vi "2D_Jacobi_eigenvalue_algorithm_v2.vi"() -> (3 "Jacobi Eigvals":dbl[](array[numeric]))   [LabVIEW 2020]
uses:
  <vilib>/Analysis/baseanly.llb/Real A x B.vi
  <vilib>/Analysis/Matrix/Numeric/Conversions/Array To Matrix - RA2.vi
  <vilib>/Analysis/Matrix/Numeric/Conversions/Matrix To Array - RM.vi
  <vilib>/Analysis/7linalg.llb/Real Eigenvalues and Vectors.vi
  <vilib>/Analysis/Matrix/NI_Matrix.lvlib
  <vilib>/Analysis/NI_AALBase.lvlib
  <vilib>/Analysis/NI_AALPro.lvlib
panel:
  out "A":dbl[][](array[numeric])
  out "summ of error":dbl
  out "LabVIEW eigvals":dbl[](array[numeric])
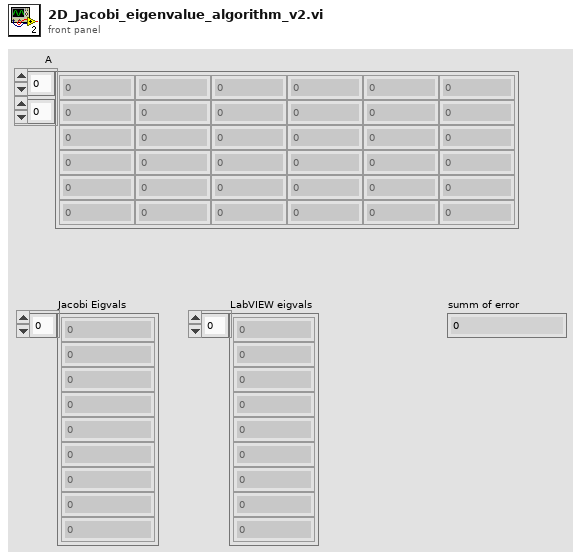
[diagram p1: front panel]
types:
  T1 = typedef "NI_Matrix.lvlib/RealMatrix.ctl" = dbl[][]
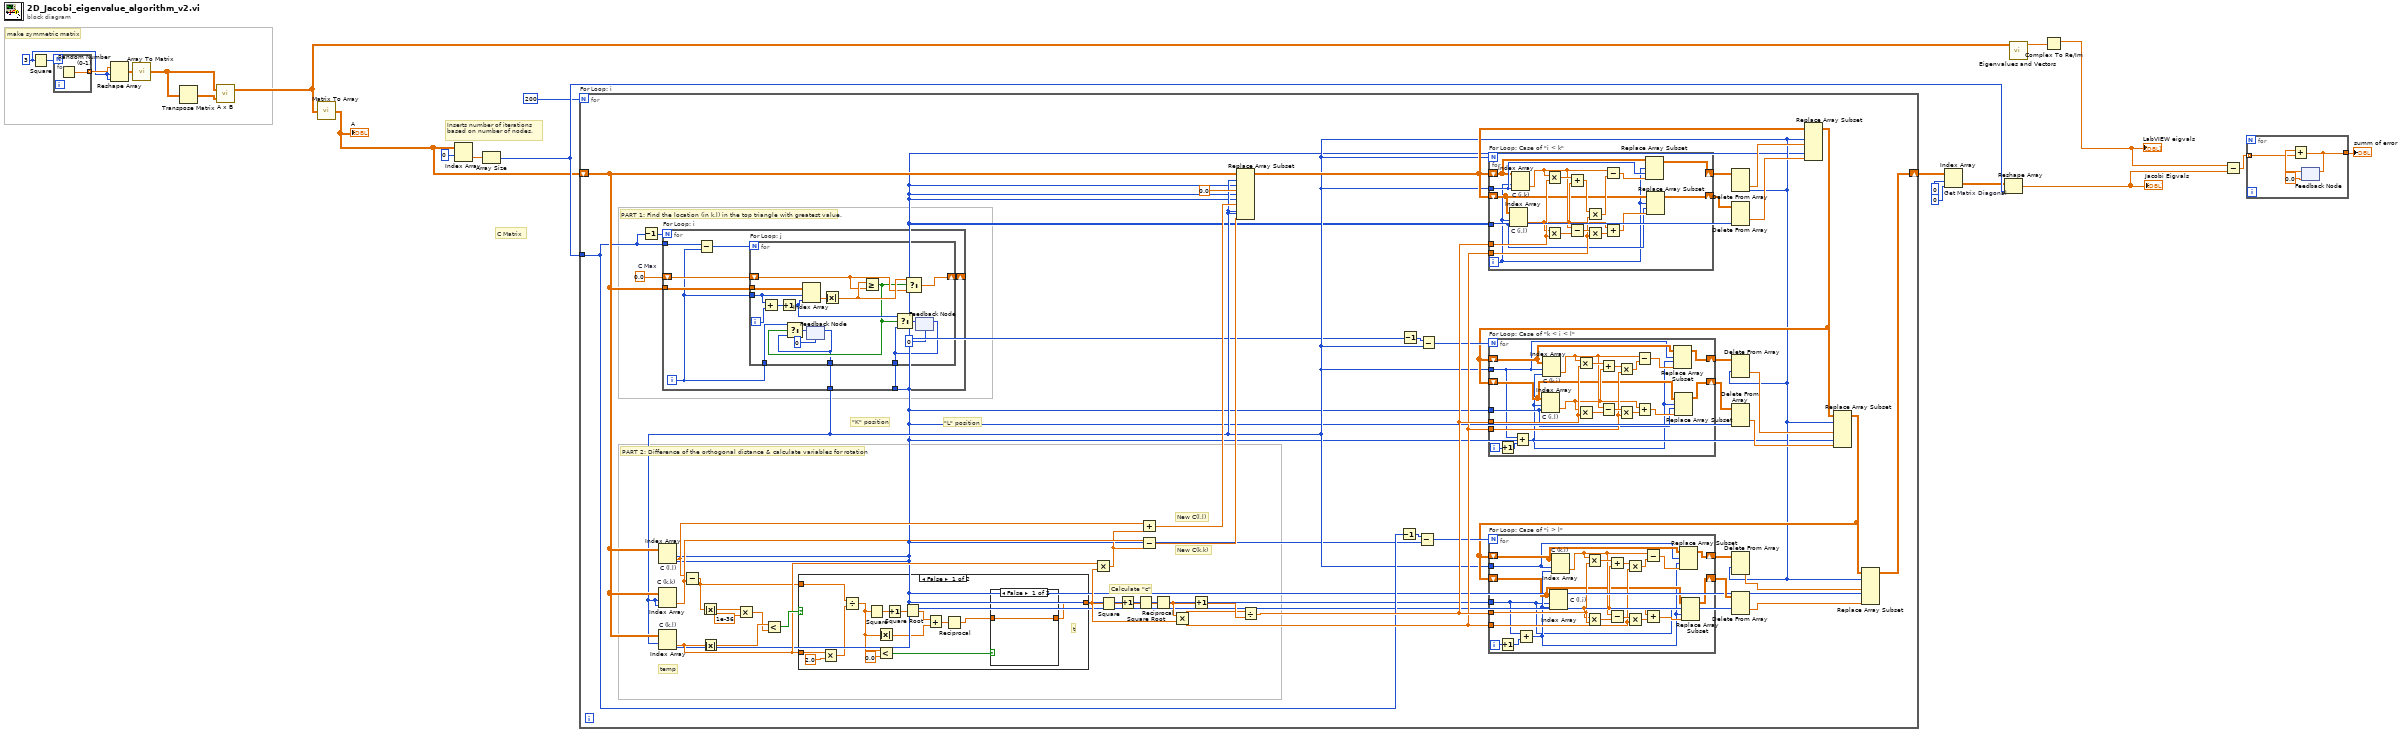
[diagram p0: block diagram]
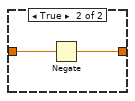
[diagram p2: hidden frame]
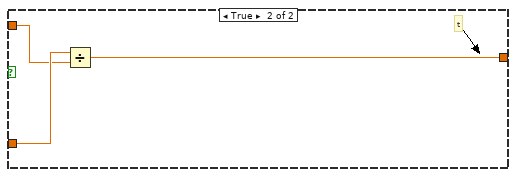
[diagram p3: hidden frame]
diagram:
  w11 = 3 ("x")
  # "make symmetric matrix"
  # "C Matrix"
  # "Inserts number of iterations\nbased on number of nodes."
  n1 = Square(x=w11) -> (x^2=w13:i32)
  n2 = for {
    N: w13 -> [_]
    tunnel: [w22] -> w12 mode=indexing
    n3 = Random Number (0-1)() -> (number: 0 to 1=w22:dbl)
  }
  n4 = Reshape Array(w12, w11, w11) -> (w10:dbl[][])
  n5 = call-poly <vilib>:"Array To Matrix.vi"("Real 2D Array"=w10) -> ("Real Matrix"=w9:T1)
  n6 = Transpose Matrix(1:w9) -> (0:w8:T1)
  n7 = call-poly <vilib>:"A x B.vi"("B"=w8, "A"=w9) -> ("A x B"=w2:T1)  [unwired: 1 out]
  n8 = call-poly <vilib>:"Matrix To Array.vi"("Real Matrix"=w2) -> ("Real 2D Array"=w1:dbl[][])
  "A" <- w1
  n9 = Index Array(array=w1, index (row)=0) -> (element=w14:dbl[])  [unwired: 1 in]
  n10 = Array Size(array=w14) -> (size(s)=w20:i32)
  n11 = for "For Loop: i" {
    N: 200 ("Max Rotation") -> [_]
    tunnel: w20 -> [w25]
    shift-right: [w29] -> w21
    shift-left: w1 -> [w47]
    w68 = 0.0  # C Max
    # "\"L\" position"
    # "\"K\" position"
    # "PART 2: Difference of the orthogonal distance & calculate variables for rotation"
    # "PART 1: Find the location (in k,l) in the top triangle with greatest value."
    # "New C(l,l)"
    # "New C(k,k)"
    # "temp"
    # "Calculate \"c\""
    n12 = Decrement(x=w25) -> (x-1=w69:i32)
    n13 = for "For Loop: i" {
      N: w69 -> [_]
      tunnel: w47 -> [w158]
      tunnel: w25 -> [w151]
      shift-right: [w156] -> _
      shift-left: w68 -> [w154]
      tunnel: [w155] -> w23
      tunnel: [w153] -> w24
      i -> [w152]
      n14 = Subtract(x=w151, y=w152) -> (x-y=w157:i32)
      n15 = for "For Loop: j" {
        N: w157 -> [_]
        tunnel: w158 -> [w174]
        tunnel: w152 -> [w171]
        shift-right: [w168] -> w156
        shift-left: w154 -> [w169]
        tunnel: [w165] -> w155
        tunnel: [w162] -> w153
        tunnel: w152 -> [w161]
        i -> [w173]
        n16 = Add(x=w171, y=w173) -> (x+y=w172:i32)
        n17 = Increment(x=w172) -> (x+1=w167:i32)
        n18 = Index Array(array=w174, index (row)=w171, index (col)=w167) -> (element=w175:dbl)
        n19 = feedback #1(0) -> (w162:i32)
        n20 = Absolute Value(x=w175) -> (abs(x)=w170:dbl)
        n21 = Greater Or Equal?(x=w170, y=w169) -> (x >= y?=w163:bool)
        n22 = Select(t=w161, s=w163, f=w162) -> (s? t:f=w164:i32)
        n23 = feedback-in #1(w164) -> ()
        n24 = Select(t=w170, s=w163, f=w169) -> (s? t:f=w168:dbl)
        n25 = feedback #2(0) -> (w165:i32)
        n26 = Select(t=w167, s=w163, f=w165) -> (s? t:f=w166:i32)
        n27 = feedback-in #2(w166) -> ()
      }
    }
    n28 = Index Array "C (l,l)"(array=w47, index (row)=w23, index (col)=w23) -> (element=w53:dbl)
    n29 = Index Array "C (k,k)"(array=w47, index (row)=w24, index (col)=w24) -> (element=w57:dbl)
    n30 = Index Array "C (k,l)"(array=w47, index (row)=w24, index (col)=w23) -> (element=w56:dbl)
    n31 = Subtract(x=w53, y=w57) -> (x-y=w48:dbl)
    n32 = Absolute Value(x=w48) -> (abs(x)=w65:dbl)
    n33 = Absolute Value(x=w56) -> (abs(x)=w67:dbl)
    n34 = Multiply(x=w65, y=1e-36 ("x")) -> (x*y=w66:dbl)
    n35 = Less?(x=w67, y=w66) -> (x < y?=w63:bool)
    n36 = case shown="False" w63 {
      tunnel: w56 -> [w144 w150]
      tunnel: w48 -> [w141 w149]
      tunnel: [w131 w148] -> w55
      frame False {
        # "t"
        n37 = Multiply(x=w144, y=2.0) -> (x*y=w142:dbl)
        n38 = Divide(x=w141, y=w142) -> (x/y=w135:dbl)
        n39 = Square(x=w135) -> (x^2=w139:dbl)
        n40 = Absolute Value(x=w135) -> (abs(x)=w140:dbl)
        n41 = Less?(x=w135, y=0.0) -> (x < y?=w133:bool)
        n42 = Increment(x=w139) -> (x+1=w138:dbl)
        n43 = Square Root(x=w138) -> (sqrt(x)=w137:dbl)
        n44 = Add(x=w137, y=w140) -> (x+y=w136:dbl)
        n45 = Reciprocal(x=w136) -> (1/x=w132:dbl)
        n46 = case shown="False" w133 {
          tunnel: w132 -> [w145 w147]
          tunnel: [w145 w146] -> w131
          frame False {
          }
          frame True {
            n47 = Negate(x=w147) -> (-x=w146:dbl)
          }
        }
      }
      frame True {
        # "t"
        n48 = Divide(x=w150, y=w149) -> (x/y=w148:dbl)
      }
    }
    n49 = Multiply(x=w56, y=w55) -> (x*y=w54:dbl)
    n50 = Square(x=w55) -> (x^2=w62:dbl)
    n51 = Increment(x=w62) -> (x+1=w61:dbl)
    n52 = Square Root(x=w61) -> (sqrt(x)=w60:dbl)
    n53 = Add(x=w53, y=w54) -> (x+y=w45:dbl)
    n54 = Subtract(x=w57, y=w54) -> (x-y=w46:dbl)
    n55 = Reciprocal(x=w60) -> (1/x=w59:dbl)
    n56 = Multiply(x=w59, y=w55) -> (x*y=w51:dbl)
    n57 = Increment(x=w59) -> (x+1=w58:dbl)
    n58 = Replace Array Subset(array=w47, new element #1=0.0 ("new element/subarray"), index (row) #1=w24, index (col) #1=w23, new element #2=w45, index (row) #2=w23, index (col) #2=w23, new element #3=w46, index (row) #3=w24, index (col) #3=w24) -> (w40:dbl[][])
    n59 = Divide(x=w51, y=w58) -> (x/y=w52:dbl)
    n60 = Decrement(x=w25) -> (x-1=w26:i32)
    n61 = Decrement(x=w23) -> (x-1=w27:i32)
    n62 = Subtract(x=w26, y=w23) -> (x-y=w50:i32)
    n63 = Subtract(x=w27, y=w24) -> (x-y=w49:i32)
    n64 = for "For Loop: Case of \"i < k\"" {
      N: w24 -> [_]
      tunnel: w52 -> [w127]
      tunnel: w51 -> [w124]
      tunnel: w24 -> [w119]
      tunnel: w23 -> [w114]
      shift-right: [w117] -> w44
      shift-left: w40 -> [w118]
      shift-right: [w113] -> w43
      shift-left: w40 -> [w116]
      i -> [w112]
      n65 = Index Array "C (i,l)"(array=w116, index (row)=w112, index (col)=w114) -> (element=w121:dbl)
      n66 = Index Array "C (i,k)"(array=w118, index (row)=w112, index (col)=w119) -> (element=w122:dbl)
      n67 = Multiply(x=w122, y=w127) -> (x*y=w130:dbl)
      n68 = Multiply(x=w121, y=w127) -> (x*y=w126:dbl)
      n69 = Add(x=w130, y=w121) -> (x+y=w129:dbl)
      n70 = Subtract(x=w122, y=w126) -> (x-y=w125:dbl)
      n71 = Multiply(x=w129, y=w124) -> (x*y=w128:dbl)
      n72 = Multiply(x=w125, y=w124) -> (x*y=w123:dbl)
      n73 = Subtract(x=w122, y=w128) -> (x-y=w120:dbl)
      n74 = Add(x=w121, y=w123) -> (x+y=w115:dbl)
      n75 = Replace Array Subset(array=w118, new element=w120, index (row)=w112, index (col)=w119) -> (w117:dbl[][])
      n76 = Replace Array Subset(array=w116, new element=w115, index (row)=w112, index (col)=w114) -> (w113:dbl[][])
    }
    n77 = Delete From Array(array=w44, index (col)=w24) -> (deleted portion=w41:dbl[])  [unwired: 2 in, 1 out]
    n78 = Delete From Array(array=w43, index (col)=w23) -> (deleted portion=w42:dbl[])  [unwired: 2 in, 1 out]
    n79 = Replace Array Subset(array=w40, new element #1=w41, index (col) #1=w24, new element #2=w42, index (col) #2=w23) -> (w37:dbl[][])  [unwired: 2 in]
    n80 = for "For Loop: Case of \"k < i < l\"" {
      N: w49 -> [_]
      tunnel: w52 -> [w108]
      tunnel: w51 -> [w105]
      tunnel: w23 -> [w95]
      tunnel: w24 -> [w93]
      shift-right: [w99] -> w36
      shift-left: w37 -> [w101]
      shift-right: [w98] -> w35
      shift-left: w37 -> [w97]
      i -> [w92]
      n81 = Increment(x=w92) -> (x+1=w91:i32)
      n82 = Add(x=w93, y=w91) -> (x+y=w94:i32)
      n83 = Index Array "C (i,l)"(array=w97, index (row)=w94, index (col)=w95) -> (element=w102:dbl)
      n84 = Index Array "C (k,i)"(array=w101, index (row)=w93, index (col)=w94) -> (element=w103:dbl)
      n85 = Multiply(x=w103, y=w108) -> (x*y=w111:dbl)
      n86 = Multiply(x=w102, y=w108) -> (x*y=w107:dbl)
      n87 = Add(x=w111, y=w102) -> (x+y=w110:dbl)
      n88 = Subtract(x=w103, y=w107) -> (x-y=w106:dbl)
      n89 = Multiply(x=w110, y=w105) -> (x*y=w109:dbl)
      n90 = Multiply(x=w106, y=w105) -> (x*y=w104:dbl)
      n91 = Subtract(x=w103, y=w109) -> (x-y=w100:dbl)
      n92 = Add(x=w102, y=w104) -> (x+y=w96:dbl)
      n93 = Replace Array Subset(array=w101, new element=w100, index (row)=w93, index (col)=w94) -> (w99:dbl[][])
      n94 = Replace Array Subset(array=w97, new element=w96, index (row)=w94, index (col)=w95) -> (w98:dbl[][])
    }
    n95 = Delete From Array(array=w36, index (row)=w24) -> (deleted portion=w38:dbl[])  [unwired: 2 in, 1 out]
    n96 = Delete From Array(array=w35, index (col)=w23) -> (deleted portion=w39:dbl[])  [unwired: 2 in, 1 out]
    n97 = Replace Array Subset(array=w37, new element #1=w38, index (row) #1=w24, new element #2=w39, index (col) #2=w23) -> (w34:dbl[][])  [unwired: 2 in]
    n98 = for "For Loop: Case of \"i > l\"" {
      N: w50 -> [_]
      tunnel: w52 -> [w87]
      tunnel: w51 -> [w84]
      tunnel: w24 -> [w78]
      tunnel: w23 -> [w72]
      shift-right: [w77] -> w33
      shift-left: w34 -> [w80]
      shift-right: [w75] -> w32
      shift-left: w34 -> [w76]
      i -> [w71]
      n99 = Increment(x=w71) -> (x+1=w70:i32)
      n100 = Add(x=w72, y=w70) -> (x+y=w73:i32)
      n101 = Index Array "C (l,i)"(array=w76, index (row)=w72, index (col)=w73) -> (element=w81:dbl)
      n102 = Index Array "C (k,i)"(array=w80, index (row)=w78, index (col)=w73) -> (element=w82:dbl)
      n103 = Multiply(x=w82, y=w87) -> (x*y=w90:dbl)
      n104 = Multiply(x=w81, y=w87) -> (x*y=w86:dbl)
      n105 = Add(x=w90, y=w81) -> (x+y=w89:dbl)
      n106 = Subtract(x=w82, y=w86) -> (x-y=w85:dbl)
      n107 = Multiply(x=w89, y=w84) -> (x*y=w88:dbl)
      n108 = Multiply(x=w85, y=w84) -> (x*y=w83:dbl)
      n109 = Subtract(x=w82, y=w88) -> (x-y=w79:dbl)
      n110 = Add(x=w81, y=w83) -> (x+y=w74:dbl)
      n111 = Replace Array Subset(array=w80, new element=w79, index (row)=w78, index (col)=w73) -> (w77:dbl[][])
      n112 = Replace Array Subset(array=w76, new element=w74, index (row)=w72, index (col)=w73) -> (w75:dbl[][])
    }
    n113 = Delete From Array(array=w33, index (row)=w24) -> (deleted portion=w31:dbl[])  [unwired: 2 in, 1 out]
    n114 = Delete From Array(array=w32, index (row)=w23) -> (deleted portion=w30:dbl[])  [unwired: 2 in, 1 out]
    n115 = Replace Array Subset(array=w34, new element #1=w31, index (row) #1=w24, new element #2=w30, index (row) #2=w23) -> (w29:dbl[][])  [unwired: 2 in]
  }
  n116 = Index Array "Get Matrix Diagonal"(array=w21, index (row)=0, index (col)=0) -> (element=w18:dbl[][])
  n117 = Reshape Array(w18, w20) -> (w5:dbl[])
  "Jacobi Eigvals" <- w5
  n118 = call-poly <vilib>:"Eigenvalues and Vectors.vi"("Input Matrix"=w2) -> ("Eigenvalues"=w7:cdb[])  [unwired: 2 in, 2 out]
  n119 = Complex To Re/Im(x + iy=w7) -> (x=w6:dbl[])  [unwired: 1 out]
  "LabVIEW eigvals" <- w6
  n120 = Subtract(x=w6, y=w5) -> (x-y=w4:dbl[])
  n121 = for {
    tunnel: w4 -> [w178] mode=indexing
    tunnel: [w176] -> w3
    n122 = feedback #3(0.0) -> (w179:dbl)
    n123 = Add(x=w179, y=w178) -> (x+y=w176:dbl)
    n124 = feedback-in #3(w176) -> ()
  }
  "summ of error" <- w3
